vi "PWM.vi"(0 "Echo Sebelum":bool, 1 "Echo Saat Ini":bool, 2 "Tick Saat Ini":i32, 3 "PWM Input Saat Ini":i32, 4 "PWM Input Sebelum":i32) -> (5 "PWM Output Saat Ini":i32, 6 "PWM Output":i32)   [LabVIEW 2019]
doc: "The myRIO Project template acquires acceleration data from the onboard accelerometer and displays the changes of acceleration values in a waveform chart."
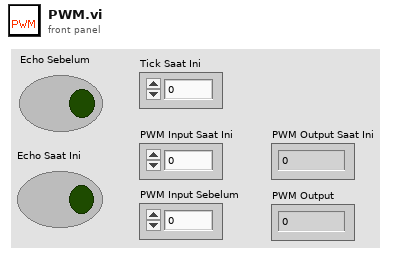
[diagram p1: front panel]
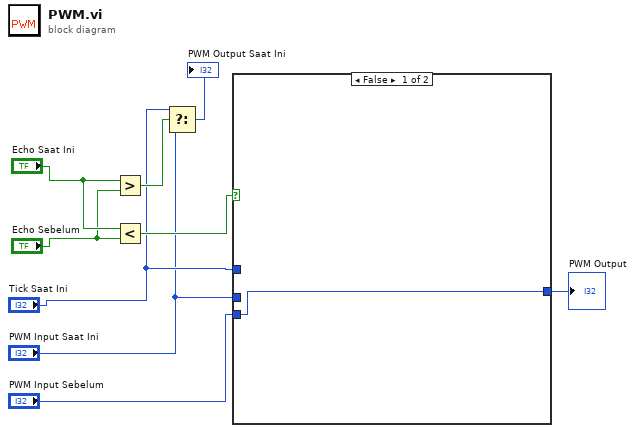
[diagram p0: block diagram]
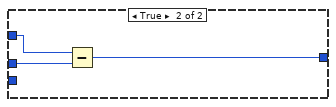
[diagram p2: hidden frame]
diagram:
  n1 = Greater?(x="Echo Saat Ini", y="Echo Sebelum") -> (0:w6:bool)
  n2 = Less?(x="Echo Saat Ini", y="Echo Sebelum") -> (x < y?=w7:bool)
  n3 = Select(t="Tick Saat Ini", s=w6, f="PWM Input Saat Ini") -> (s? t:f=→"PWM Output Saat Ini":i32)
  n4 = case shown="False" w7 {
    tunnel: "PWM Input Sebelum" -> [w10 _]
    tunnel: "Tick Saat Ini" -> [_ w13]
    tunnel: "PWM Input Saat Ini" -> [_ w12]
    tunnel: [w10 w11] -> w1
    frame False {
    }
    frame True {
      n5 = Subtract(x=w13, y=w12) -> (x-y=w11:i32)
    }
  }
  "PWM Output" <- w1
